vi "ELVIS III v1.0 Build MUX Configuration AI Block.vi"(11 "AI (N Samples) Channels List":T4) -> (3 "Channel Reservation Info":T1)   [LabVIEW 2021]
uses:
  <vilib>/myRIO/Common/Instrument Driver Framework/myRIO v1.0/AI Block/typedefs/AI Block Channels List.ctl
  <vilib>/myRIO/Common/Instrument Driver Framework/myRIO v1.0/AI Block/typedefs/AI Block Channels Enum.ctl
  <vilib>/myRIO/Common/Instrument Driver Framework/ELVIS III v1.0/Resource Manager/typedefs/ELVIS III v1.0 Channel Reservation List.ctl
  <vilib>/myRIO/Common/Instrument Driver Framework/ELVIS III v1.0/Resource Manager/typedefs/ELVIS III v1.0 Channel Reservation Info.ctl
  <vilib>/myRIO/Common/Instrument Driver Framework/ELVIS III v1.0/Resource Manager/typedefs/ELVIS III v1.0 Connector List.ctl
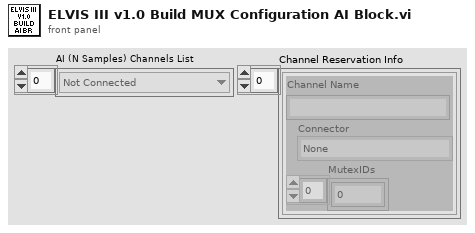
[diagram p1: front panel]
types:
  T1 = typedef "ELVIS III v1.0 Channel Reservation List.ctl" = T2[]
  T2 = typedef "ELVIS III v1.0 Channel Reservation Info.ctl" = cluster{"Channel Name":string, "Connector":T3, "MutexIDs":u32[]}
  T3 = typedef "ELVIS III v1.0 Connector List.ctl" = enum32{"None", "ConnectorA", "ConnectorB"}
  T4 = typedef "AI Block Channels List.ctl" = T5[]
  T5 = typedef "AI Block Channels Enum.ctl" = enum16{"Not Connected", "A/AI0 (N Samples)", "A/AI1 (N Samples)", "A/AI2 (N Samples)", "A/AI3 (N Samples)", "A/AI4 (N Samples)", "A/AI5 (N Samples)", "A/AI6 (N Samples)", "A/AI7 (N Samples)", "A/AI0 (DIFF N Samples)", "A/AI1 (DIFF N Samples)", "A/AI2 (DIFF N Samples)", "A/AI3 (DIFF N Samples)", "B/AI0 (N Samples)", "B/AI1 (N Samples)", "B/AI2 (N Samples)", "B/AI3 (N Samples)", "B/AI4 (N Samples)", "B/AI5 (N Samples)", "B/AI6 (N Samples)", "B/AI7 (N Samples)", "B/AI0 (DIFF N Samples)", "B/AI1 (DIFF N Samples)", "B/AI2 (DIFF N Samples)", "B/AI3 (DIFF N Samples)"}
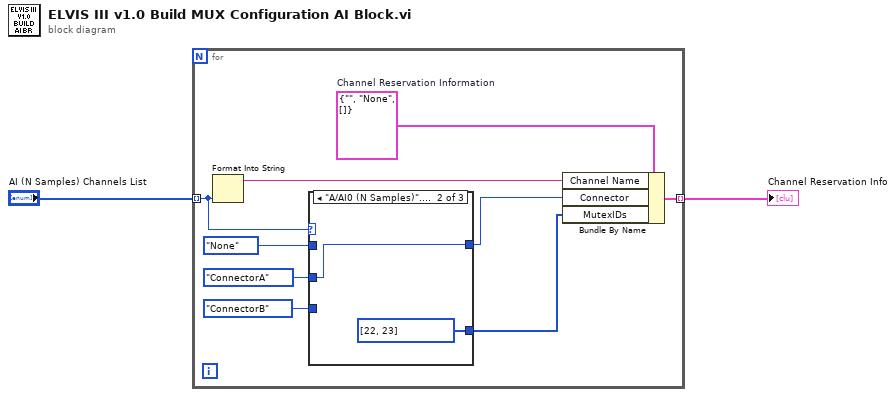
[diagram p0: block diagram]
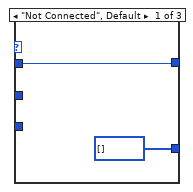
[diagram p2: hidden frame]
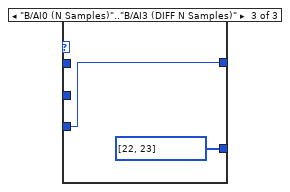
[diagram p3: hidden frame]
diagram:
  n1 = for {
    tunnel: "AI (N Samples) Channels List" -> [w8] mode=indexing
    tunnel: [w9] -> w1 mode=indexing
    w11 = T2 {"Channel Name"="", "Connector"=enum."None", "MutexIDs"=[]}  # Channel Reservation Information
    n2 = Format Into String(w8) -> (resulting string=w10:string)  [unwired: 3 in, 1 out]
    n3 = case shown="\"A/AI0 (N Samples)\"..\"A/AI3 (DIFF N Samples)\"" w8 {
      tunnel: [u32[] [] ("MutexIDs") u32[] [22, 23] ("MutexIDs") u32[] [22, 23] ("MutexIDs")] -> w7
      tunnel: ELVIS_III_v1.0_Connector_List."None" ("Connector") -> [w13 _ _]
      tunnel: [w13 w15 w16] -> w5
      tunnel: ELVIS_III_v1.0_Connector_List."ConnectorA" ("Connector") -> [_ w15 _]
      tunnel: ELVIS_III_v1.0_Connector_List."ConnectorB" ("Connector") -> [_ _ w16]
      frame "Not Connected", Default {
      }
      frame "A/AI0 (N Samples)".."A/AI3 (DIFF N Samples)" {
      }
      frame "B/AI0 (N Samples)".."B/AI3 (DIFF N Samples)" {
      }
    }
    n4 = Bundle By Name(cluster=w11, "Channel Name"=w10, "Connector"=w5, "MutexIDs"=w7) -> (w9:T2)
  }
  "Channel Reservation Info" <- w1
